vi "update CD name in XML file.vi"(8 "error in":errorcluster, 11 "custom device path":path=path "C:/Users/nitest/Documents/LabVIEW Data") -> (0 "error out":errorcluster, 3 "custom device path out":path=path "C:/Users/nitest/Documents/LabVIEW Data")   [LabVIEW 2020, in "Template Tool.lvlib"]
uses:
  Template Tool.lvlib
  NationalInstruments.VeriStand.XMLReader
  Template Tool Global.vi
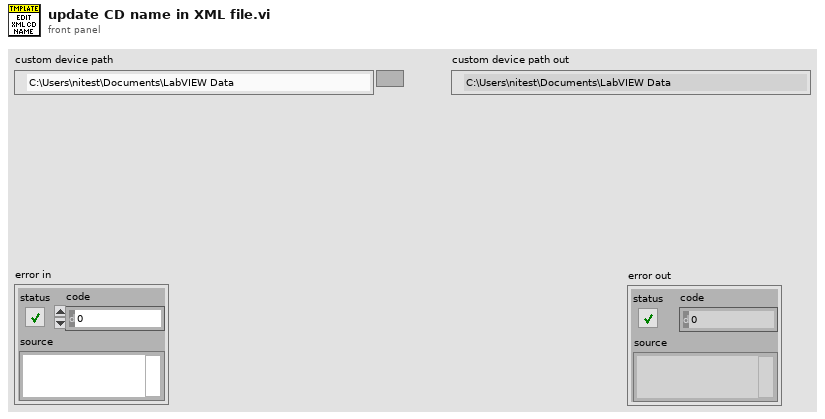
[diagram p1: front panel]
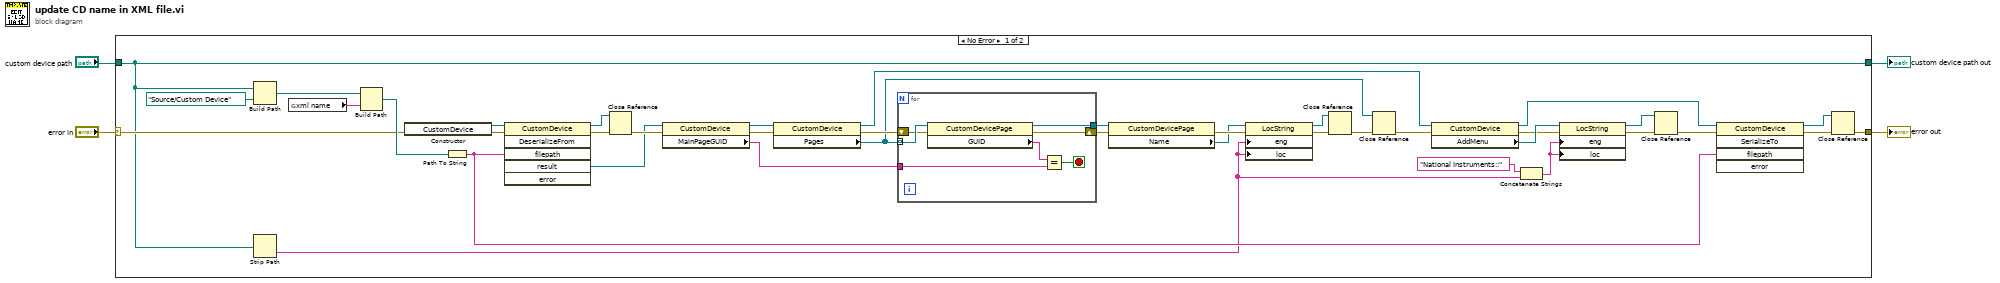
[diagram p0: block diagram]
diagram:
  n1 = case shown="No Error" "error in" {
    selector: "error in" -> [w18 w52]
    tunnel: "custom device path" -> [w17 w51]
    tunnel: [w24 w52] -> w3
    tunnel: [w17 w51] -> w1
    frame No Error {
      n2 = Build Path(base path=w17, name or relative path=path "Source/Custom Device") -> (appended path=w42:path)
      n3 = Strip Path(path=w17) -> (name=w11:string)  [unwired: 1 out]
      n4 = global read "Template Tool Global.vi" "xml name"() -> (w16:string)
      n5 = Build Path(base path=w42, name or relative path=w16) -> (appended path=w37:path)
      n6 = constructor class="CustomDevice"(error in=w18) -> (reference out=w39:refnum<k24>, error out=w38:errorcluster)  [unwired: 2 in, 1 out]
      n7 = Path To String(path=w37) -> (string=w19:string)
      n8 = invoke class="CustomDevice" method="DeserializeFrom"(reference=w39, error in=w38, "filepath"=w19) -> (reference out=w41:refnum<k24>, error out=w40:errorcluster, "result"=w33:refnum<k24>)  [unwired: 3 in, 3 out]
      n9 = Close Reference(reference=w41, error in (no error)=w40) -> (error out=w34:errorcluster)
      n10 = property class="CustomDevice"(reference=w33, error in=w34) -> (reference out=w32:refnum<k24>, error out=w31:errorcluster, "MainPageGUID"=w29:string)
      n11 = property class="CustomDevice"(reference=w32, error in=w31) -> (reference out=w6:refnum<k24>, error out=w30:errorcluster, "Pages"=w23:refnum<k24>[])
      n12 = for {
        tunnel: w23 -> [w50] mode=indexing
        shift-right: [w48] -> w28
        shift-left: w30 -> [w49]
        tunnel: w29 -> [w46]
        tunnel: [w45] -> w27
        stop <- w44 stop-if-true
        n13 = property class="CustomDevicePage"(reference=w50, error in=w49) -> (reference out=w45:refnum<k24>, error out=w48:errorcluster, "GUID"=w47:string)
        n14 = Equal?(x=w47, y=w46) -> (x = y?=w44:bool)
      }
      n15 = property class="CustomDevicePage"(reference=w27, error in=w28) -> (error out=w26:errorcluster, "Name"=w25:refnum<k24>)  [unwired: 1 out]
      n16 = property class="LocString"(reference=w25, error in=w26, "eng"=w11, "loc"=w11) -> (reference out=w22:refnum<k24>, error out=w21:errorcluster)
      n17 = Close Reference(reference=w22, error in (no error)=w21) -> (error out=w20:errorcluster)
      n18 = Close Reference(reference=w23, error in (no error)=w20) -> (error out=w15:errorcluster)
      n19 = property class="CustomDevice"(reference=w6, error in=w15) -> (reference out=w5:refnum<k24>, error out=w13:errorcluster, "AddMenu"=w14:refnum<k24>)
      n20 = Concatenate Strings("National Instruments::" ("name"), w11) -> (w10:string)
      n21 = property class="LocString"(reference=w14, error in=w13, "eng"=w10, "loc"=w10) -> (reference out=w9:refnum<k24>, error out=w8:errorcluster)
      n22 = Close Reference(reference=w9, error in (no error)=w8) -> (error out=w7:errorcluster)
      n23 = invoke class="CustomDevice" method="SerializeTo"(reference=w5, error in=w7, "filepath"=w19) -> (reference out=w36:refnum<k24>, error out=w35:errorcluster)  [unwired: 2 in, 3 out]
      n24 = Close Reference(reference=w36, error in (no error)=w35) -> (error out=w24:errorcluster)
    }
    frame Error {
    }
  }
  "error out" <- w3
  "custom device path out" <- w1
